vi "Stop Core.vi"(10 "final error code":i32, 11 "Measure Object in":refnum<class "TDMS Properties.lvclass">) -> (3 "Measure Object out":refnum<class "TDMS Properties.lvclass">)   [LabVIEW 2021, in "TDMS Properties.lvclass"]
doc: "(<B>Filename</B>: Actor Framework.lvlib:Actor.lvclass:Stop Core.vi)\n\nDefines what the actor does before it stops. Use the <B>final error code</B> input to determine whether the actor shut down in response to an error.\n\nBy default, this method does nothing. A descendant class may override it to define behavior, such as shutting down any processes the actor initiated in its override of the Actor Core method."
uses:
  TDMS Properties.lvclass
  TDMS Properties.lvclass/TDMS Properties.ctl
  Template Module/Template Module.lvclass
  <vilib>/ActorFramework/Actor/Actor.lvclass
  Controllers/Application Controller Messages/Plot Closed Msg/Plot Closed Msg.lvclass
  C:/GitHub/LabActor/Template Module/Template Module.lvclass
  C:/Program Files/National Instruments/LabVIEW 2021/vi.lib/ActorFramework/Actor/Actor.lvclass
  C:/GitHub/LabActor/Plots/TDMS Properties/TDMS Properties.lvclass
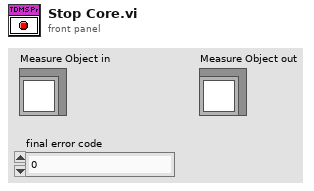
[diagram p1: front panel]
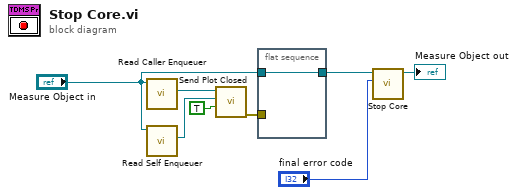
[diagram p0: block diagram]
diagram:
  n1 = call <vilib>:"Read Caller Enqueuer.vi"("Actor"="Measure Object in") -> ("Caller Enqueuer"=w6:refnum<class "Message Enqueuer.lvclass">)  [unwired: 10 in]
  n2 = call <vilib>:"Read Self Enqueuer.vi"("Actor"="Measure Object in") -> ("Self Enqueuer"=w5:refnum<class "Message Enqueuer.lvclass">)  [unwired: 10 in]
  n3 = call "Send Plot Closed.vi"("Not a plot"=TRUE, "Closed plot"=w5, "Message Enqueuer"=w6) -> ("error out"=w1:errorcluster)  [unwired: 7 in, 1 out]
  n4 = flat-sequence {
    tunnel: "Measure Object in" -> [w9]
    tunnel: [w9] -> w2
    tunnel: w1 -> [_]
    frame #0 {
    }
  }
  n5 = call-parent "Stop Core.vi"("final error code"="final error code", "Measure Object in"=w2) -> ("Measure Object out"=→"Measure Object out":refnum<class "TDMS Properties.lvclass">)  [unwired: 9 in]
